vi "hw6p5_hickey.vi"() -> ()   [LabVIEW 2014]
uses:
  <vilib>/gmath/SpecialFunctions.llb/Error Function.vi
  <vilib>/imath/engines/lvmath2/RunTimeEngine/Managers/WorkSpace/UID Generator.vi
  <vilib>/imath/engines/lvmath2/RunTimeEngine/RunTimeType/NIMS_RunTimeType_From StrictType (excl LVString).vi
  <instcachedir>/0/NIMS_RunTimeType_From StrictType (excl LVString)_15A5391EEA9C4AACB9955AC755B83D29.lvgen/NIMS_RunTimeType_From StrictType (excl LVString)_15A5391EEA9C4AACB9955AC755B83D29_000.vi
  <vilib>/imath/engines/lvmath2/RunTimeEngine/LocalVariableDefStatement/MC_LocalVariableDefStatement_Display.vi
  <vilib>/imath/engines/lvmath2/RunTimeEngine/Managers/SymbolTable/Clear UID.vi
  <vilib>/imath/engines/lvmath2/RunTimeEngine/NodeEndStatement/NIMS_NodeEndStatement_Output.vi
  <instcachedir>/0/NIMS_NodeEndStatement_Output_53EC0D466D134D7ABD903AC30B43404B.lvgen/NIMS_NodeEndStatement_Output_53EC0D466D134D7ABD903AC30B43404B_001.vi
  <vilib>/imath/engines/lvmath2/RunTimeEngine/ErrorHandling/NIMS_Finalize Error.vi
  <vilib>/Analysis/NI_AALPro.lvlib
  <vilib>/gmath/NI_Gmath.lvlib
  <vilib>/imath/engines/lvmath2/RunTimeEngine/Managers/SymbolTable/NIMS_WorkSpace.lvlib
panel:
  in  "# bins":i32
  in  "N":i32
  out "x histogram":T1(graph)
  out "Array":dbl[](array[numeric])
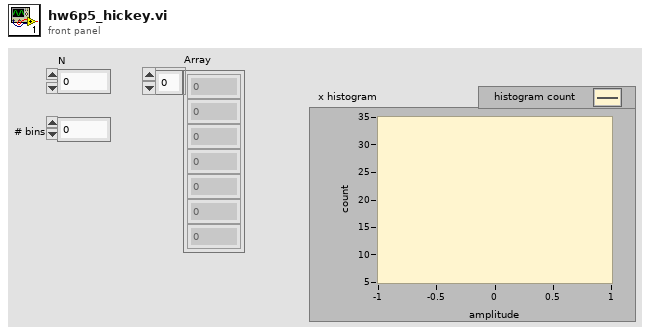
[diagram p1: front panel]
types:
  T1 = cluster{"X Values":dbl[], "Histogram: h(x)":i32[]}
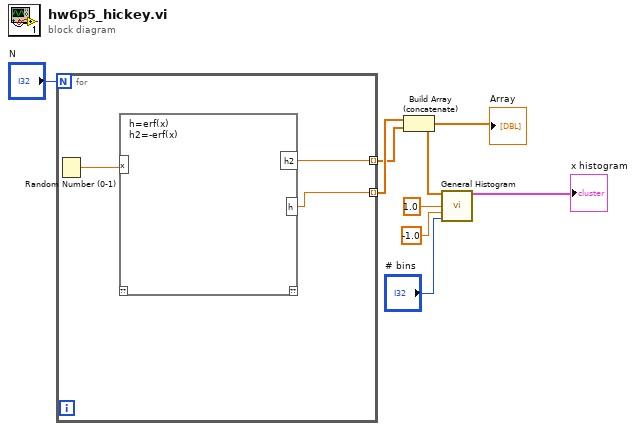
[diagram p0: block diagram]
diagram:
  n1 = for {
    N: "N" -> [_]
    tunnel: [w10] -> w3 mode=indexing
    tunnel: [w9] -> w2 mode=indexing
    n2 = Random Number (0-1)() -> (number: 0 to 1=w11:dbl)
    n3 = mathscript code="h=erf(x)\nh2=-erf(x)"("x"=w11) -> ("h"=w10:dbl, "h2"=w9:dbl)  [unwired: 1 in, 1 out]
  }
  n4 = Build Array (concatenate)(w3, w2) -> (w1:dbl[])
  "Array" <- w1
  n5 = call <vilib>:"General Histogram.vi"("X"=w1, "max"=1.0, "min"=-1.0, "# bins"="# bins") -> ("Histogram Graph"=→"x histogram":T1)  [unwired: 7 in, 4 out]
